vi "AnalysisConfig.vi"(8 "error in (no error)":errorcluster, 11 "AnalysisConfig":T6={"PortName"="WLAN_DUT0_ANT0", "PhyPort"=enum."Port5", "ExternalAtt"=0, "TriggerLevel"=-40, "NumberofChain"=1, "AcqLength"=0.0001, "MCSIndex"=7.0, "PhyType"=enum."OFDM", "Standard"=enum."802.11 n", "BW"=enum."20M", "TriggerSource"=enum."RIO0", "Freq"=5180000000.0, "LegacyDataRate"=enum."R1M"}) -> (0 "error out":errorcluster, 3 "AnalysisConfigCMD":string[](array[string])=["MEMory:TABLe:DELete:ALL", "ROUTe:RFSG:PORT:DELete:ALL", "TRIG:RFSA:WLAN:EDGE RISING", "TRIG:RFSA:WLAN:MQTime  5e-6", "ROUTe:RFSA:PORT:DEFine 'wlan_DUT0_ant0','Port0'", "CONF:RFSA:WLAN:CSEG:EATT:ALL 0", "TRIG:RFSA:WLAN:SOUR 'RF0'", "TRIG:RFSA:WLAN:THR 0", "CONF:RFSA:WLAN:NCH 0", "CONF:RFSA:WLAN:CSEG:PORT \"wlan_DUT0_ant0\"", "CONF:RFSA:WLAN:CSEG:FREQ:CENT 5", "CONF:RFSA:WLAN:BWID 0", "CONF:RFSA:WLAN:STAN A", "CONF:RFSA:WLAN:ALENgth 0", "CONF:RFSA:WLAN:PACK:MCS 0", "CONF:RFSA:WLAN:PHY DSSS", "CONF:RFSA:WLAN:ACT:ALL 1", "CONF:RFSA:WLAN:CSEG:POW:AUTO ON", "CONF:RFSA:WLAN:PACK:NSTS 1 ", "CONF:RFSA:WLAN:PACK:GINT LONG", "CONF:RFSA:WLAN:PACK:DMOD ALL", "CONF:RFSA:WLAN:PACK:PAYL:LENGth 1500", "CONF:RFSA:WLAN:MEAS:MOD:ENAB ON", "CONF:RFSA:WLAN:MEAS:MOD:OFDM:EST:COFF ON", "CONF:RFSA:WLAN:MEAS:MOD:OFDM:EST:IMP ON", "CONF:RFSA:WLAN:MEAS:MOD:OFDM:TRAC:AMPL OFF", "CONF:RFSA:WLAN:MEAS:MOD:OFDM:TRAC:CHAN OFF", "CONF:RFSA:WLAN:MEAS:MOD:OFDM:TRAC:TIME ON", "CONF:RFSA:WLAN:MEAS:MOD:OFDM:TRAC:PHAS NONE", "CONF:RFSA:WLAN:MEAS:MOD:AVER:COUN 50", "CONF:RFSA:WLAN:MEAS:MOD:OFDM:MSYM 16", "CONF:RFSA:WLAN:MEAS:SEM:ENAB ON ", "CONF:RFSA:WLAN:MEAS:SEM:AVER:COUN 3", "CONF:RFSA:WLAN:MEAS:SEM:SPAN:AUTO:ENAB ON", "CONF:RFSA:WLAN:MEAS:OBW:ENAB ON", "CONF:RFSA:WLAN:MEAS:OBW:AVER:COUN 3", "CONF:RFSA:WLAN:MEAS:TXP:ENAB ON", "CONF:RFSA:WLAN:MEAS:TXP:AVER:COUN 3"])   [LabVIEW 2015]
uses:
  PhyPort.ctl
  PhyType.ctl
  standard.ctl
  BW.ctl
  LegacyDataRate.ctl
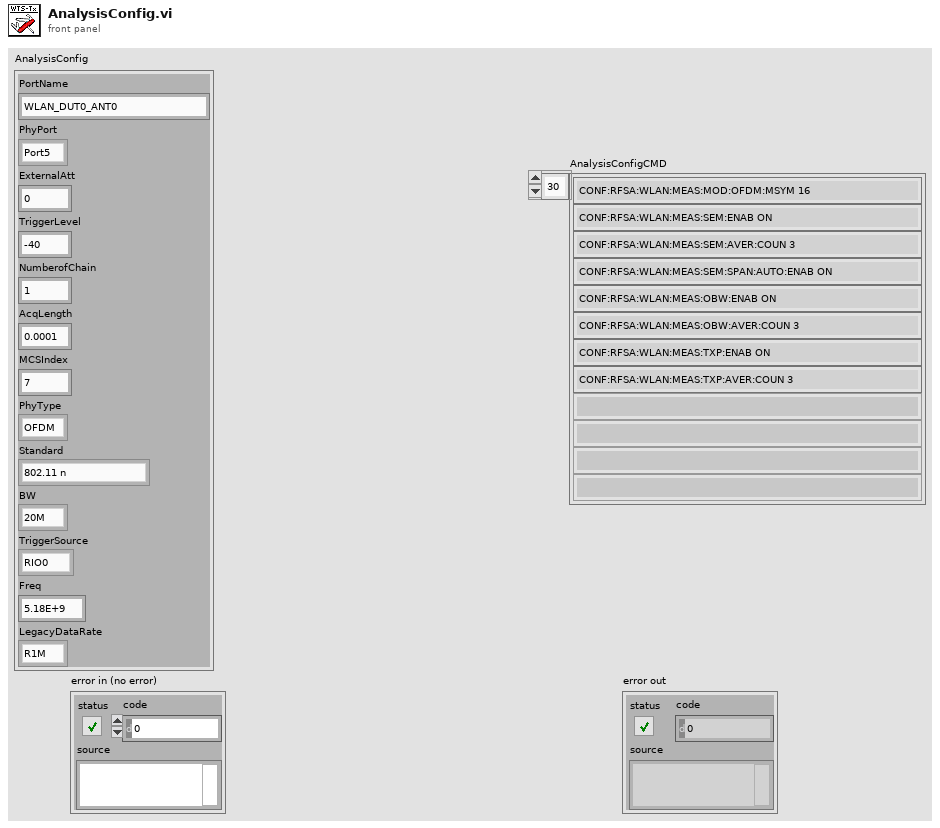
[diagram p1: front panel]
types:
  T1 = typedef "PhyPort.ctl" = enum16{"Port0", "Port1", "Port2", "Port3", "Port4", "Port5", "Port6", "Port7"}
  T2 = typedef "PhyType.ctl" = enum16{"DSSS", "OFDM", "HT", "VHT"}
  T3 = typedef "standard.ctl" = enum16{"802.11 a/g", "802.11 b/g", "802.11 g", "802.11 n", "802.11 ac"}
  T4 = typedef "BW.ctl" = enum16{"5M", "10M", "20M", "40M", "80M", "160M"}
  T5 = typedef "LegacyDataRate.ctl" = enum16{"R1M", "R2M", "R5M5", "R6M", "R9M", "R11M", "R12M", "R18M", "R24M", "R36M", "R48M", "R54M"}
  T6 = cluster{"PortName":string, "PhyPort":T1, "ExternalAtt":i32, "TriggerLevel":i32, "NumberofChain":i32, "AcqLength":dbl, "MCSIndex":dbl, "PhyType":T2, "Standard":T3, "BW":T4, "TriggerSource":enum16{"RIO0", "RIO1"}, "Freq":dbl, "LegacyDataRate":T5}
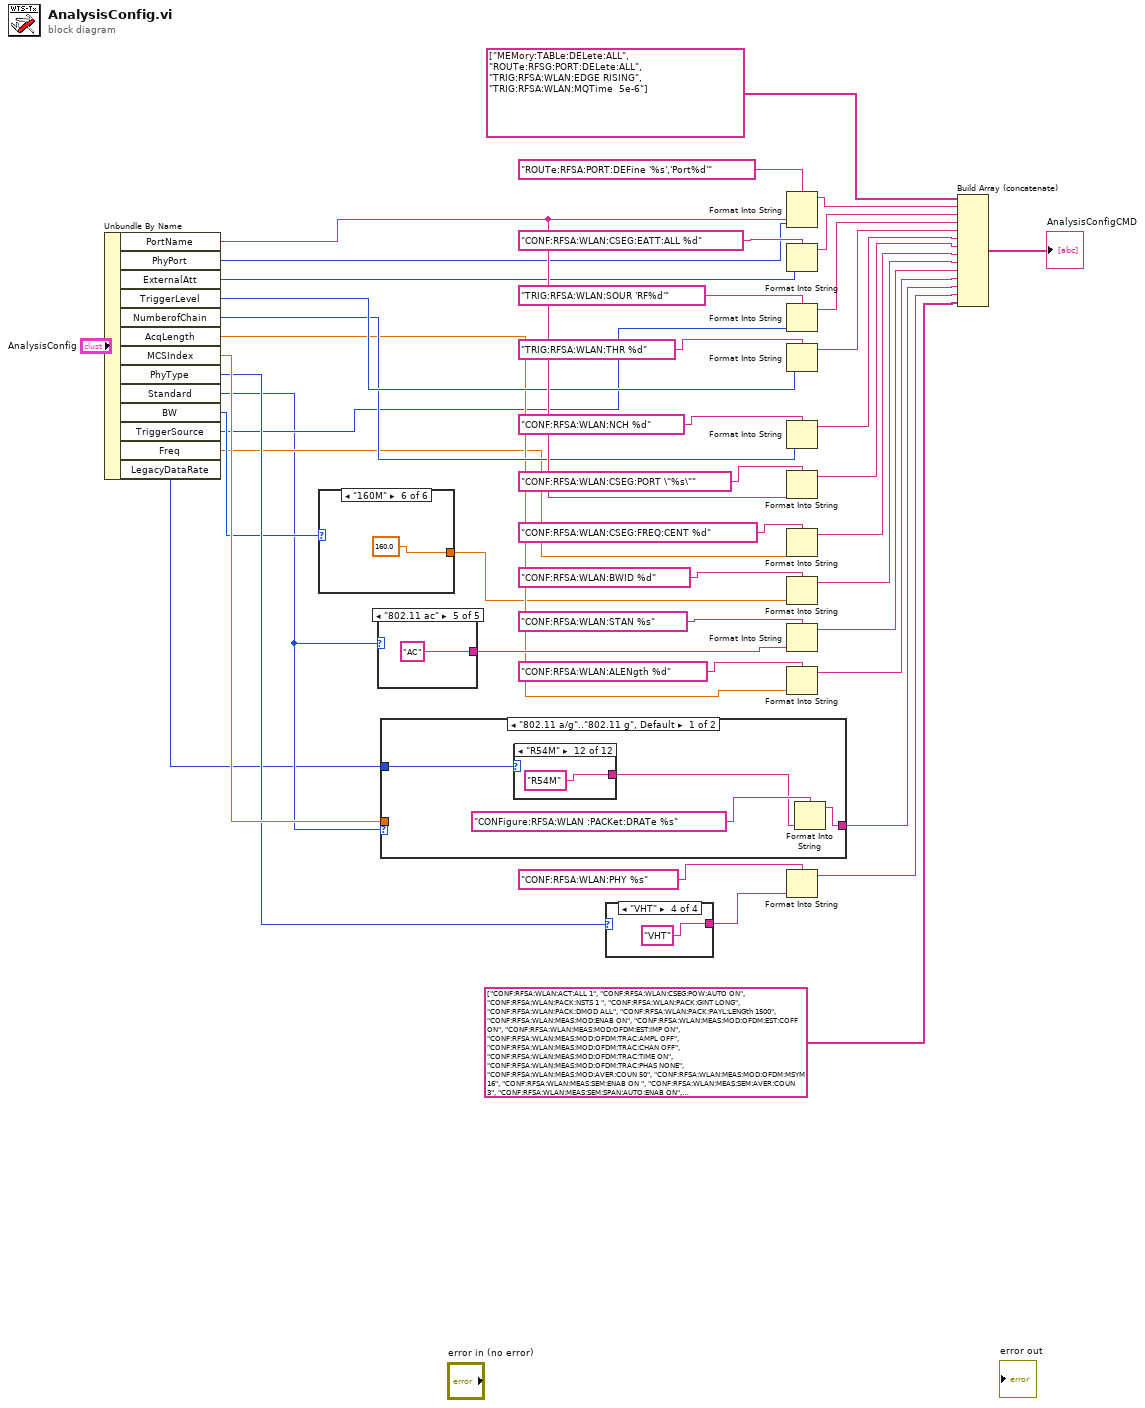
[diagram p0: block diagram]
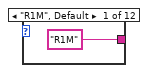
[diagram p2: hidden frame]
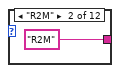
[diagram p3: hidden frame]
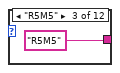
[diagram p4: hidden frame]
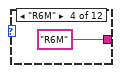
[diagram p5: hidden frame]
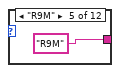
[diagram p6: hidden frame]
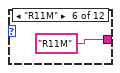
[diagram p7: hidden frame]
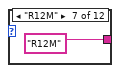
[diagram p8: hidden frame]
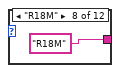
[diagram p9: hidden frame]
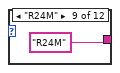
[diagram p10: hidden frame]
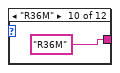
[diagram p11: hidden frame]
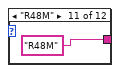
[diagram p12: hidden frame]
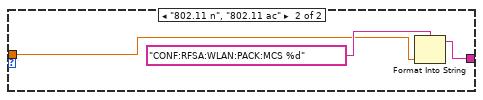
[diagram p13: hidden frame]
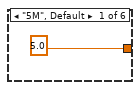
[diagram p14: hidden frame]
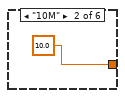
[diagram p15: hidden frame]
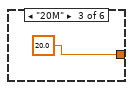
[diagram p16: hidden frame]
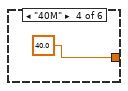
[diagram p17: hidden frame]
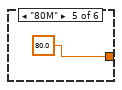
[diagram p18: hidden frame]
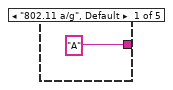
[diagram p19: hidden frame]
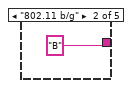
[diagram p20: hidden frame]
diagram:
  n1 = Unbundle By Name("AnalysisConfig") -> ("PortName"=w14:string, "PhyPort"=w13:T1, "ExternalAtt"=w12:i32, "TriggerLevel"=w11:i32, "NumberofChain"=w10:i32, "AcqLength"=w8:dbl, "MCSIndex"=w9:dbl, "PhyType"=w7:T2, "Standard"=w2:T3, "BW"=w6:T4, "TriggerSource"=w5:enum16{"RIO0", "RIO1"}, "Freq"=w3:dbl, "LegacyDataRate"=w1:T5)
  n2 = case shown="\"160M\"" w6 {
    tunnel: [5.0 ("Freq") 10.0 ("Freq") 20.0 ("Freq") 40.0 ("Freq") 80.0 ("Freq") 160.0 ("Freq")] -> w4
    frame "5M", Default {
    }
    frame "10M" {
    }
    frame "20M" {
    }
    frame "40M" {
    }
    frame "80M" {
    }
    frame "160M" {
    }
  }
  n3 = case shown="\"802.11 ac\"" w2 {
    tunnel: ["A" ("Standard") "B" ("Standard") "G" ("Standard") "N" ("Standard") "AC" ("Standard")] -> w16
    frame "802.11 a/g", Default {
    }
    frame "802.11 b/g" {
    }
    frame "802.11 g" {
    }
    frame "802.11 n" {
    }
    frame "802.11 ac" {
    }
  }
  n4 = case shown="\"802.11 a/g\"..\"802.11 g\", Default" w2 {
    tunnel: [w55 w72] -> w19
    tunnel: w9 -> [_ w71]
    tunnel: w1 -> [w57 _]
    frame "802.11 a/g".."802.11 g", Default {
      n5 = case shown="\"R54M\"" w57 {
        tunnel: ["R1M" "R2M" "R5M5" "R6M" "R9M" "R11M" "R12M" "R18M" "R24M" "R36M" "R48M" "R54M"] -> w56
        frame "R1M", Default {
        }
        frame "R2M" {
        }
        frame "R5M5" {
        }
        frame "R6M" {
        }
        frame "R9M" {
        }
        frame "R11M" {
        }
        frame "R12M" {
        }
        frame "R18M" {
        }
        frame "R24M" {
        }
        frame "R36M" {
        }
        frame "R48M" {
        }
        frame "R54M" {
        }
      }
      n6 = Format Into String(format string="CONFigure:RFSA:WLAN :PACKet:DRATe %s", w56) -> (resulting string=w55:string)  [unwired: 2 in, 1 out]
    }
    frame "802.11 n", "802.11 ac" {
      n7 = Format Into String(format string="CONF:RFSA:WLAN:PACK:MCS %d", w71) -> (resulting string=w72:string)  [unwired: 2 in, 1 out]
    }
  }
  n8 = case shown="\"VHT\"" w7 {
    tunnel: ["DSSS" ("PhyType") "OFDM" ("PhyType") "HT" ("PhyType") "VHT" ("PhyType")] -> w26
    frame "DSSS", Default {
    }
    frame "OFDM" {
    }
    frame "HT" {
    }
    frame "VHT" {
    }
  }
  n9 = Format Into String(format string="ROUTe:RFSA:PORT:DEFine '%s','Port%d'", w14, w13) -> (resulting string=w38:string)  [unwired: 2 in, 1 out]
  n10 = Format Into String(format string="CONF:RFSA:WLAN:CSEG:EATT:ALL %d", w12) -> (resulting string=w37:string)  [unwired: 2 in, 1 out]
  n11 = Format Into String(format string="TRIG:RFSA:WLAN:SOUR 'RF%d'", w5) -> (resulting string=w36:string)  [unwired: 2 in, 1 out]
  n12 = Format Into String(format string="TRIG:RFSA:WLAN:THR %d", w11) -> (resulting string=w35:string)  [unwired: 2 in, 1 out]
  n13 = Format Into String(format string="CONF:RFSA:WLAN:NCH %d", w10) -> (resulting string=w25:string)  [unwired: 2 in, 1 out]
  n14 = Format Into String(format string="CONF:RFSA:WLAN:CSEG:PORT \"%s\"", w14) -> (resulting string=w24:string)  [unwired: 2 in, 1 out]
  n15 = Format Into String(format string="CONF:RFSA:WLAN:CSEG:FREQ:CENT %d", w3) -> (resulting string=w23:string)  [unwired: 2 in, 1 out]
  n16 = Format Into String(format string="CONF:RFSA:WLAN:BWID %d", w4) -> (resulting string=w22:string)  [unwired: 2 in, 1 out]
  n17 = Format Into String(format string="CONF:RFSA:WLAN:STAN %s", w16) -> (resulting string=w21:string)  [unwired: 2 in, 1 out]
  n18 = Format Into String(format string="CONF:RFSA:WLAN:ALENgth %d", w8) -> (resulting string=w20:string)  [unwired: 2 in, 1 out]
  n19 = Format Into String(format string="CONF:RFSA:WLAN:PHY %s", w26) -> (resulting string=w18:string)  [unwired: 2 in, 1 out]
  n20 = Build Array (concatenate)(string[] ["MEMory:TABLe:DELete:ALL", "ROUTe:RFSG:PORT:DELete:ALL", "TRIG:RFSA:WLAN:EDGE RISING", "TRIG:RFSA:WLAN:MQTime  5e-6"], w38, w37, w36, w35, w25, w24, w23, w22, w21, w20, w19, w18, string[] ["CONF:RFSA:WLAN:ACT:ALL 1", "CONF:RFSA:WLAN:CSEG:POW:AUTO ON", "CONF:RFSA:WLAN:PACK:NSTS 1 ", "CONF:RFSA:WLAN:PACK:GINT LONG", "CONF:RFSA:WLAN:PACK:DMOD ALL", "CONF:RFSA:WLAN:PACK:PAYL:LENGth 1500", "CONF:RFSA:WLAN:MEAS:MOD:ENAB ON", "CONF:RFSA:WLAN:MEAS:MOD:OFDM:EST:COFF ON", "CONF:RFSA:WLAN:MEAS:MOD:OFDM:EST:IMP ON", "CONF:RFSA:WLAN:MEAS:MOD:OFDM:TRAC:AMPL OFF", "CONF:RFSA:WLAN:MEAS:MOD:OFDM:TRAC:CHAN OFF", "CONF:RFSA:WLAN:MEAS:MOD:OFDM:TRAC:TIME ON", "CONF:RFSA:WLAN:MEAS:MOD:OFDM:TRAC:PHAS NONE", "CONF:RFSA:WLAN:MEAS:MOD:AVER:COUN 50", "CONF:RFSA:WLAN:MEAS:MOD:OFDM:MSYM 16", "CONF:RFSA:WLAN:MEAS:SEM:ENAB ON ", "CONF:RFSA:WLAN:MEAS:SEM:AVER:COUN 3", "CONF:RFSA:WLAN:MEAS:SEM:SPAN:AUTO:ENAB ON", "CONF:RFSA:WLAN:MEAS:OBW:ENAB ON", "CONF:RFSA:WLAN:MEAS:OBW:AVER:COUN 3", "CONF:RFSA:WLAN:MEAS:TXP:ENAB ON", "CONF:RFSA:WLAN:MEAS:TXP:AVER:COUN 3", "*OPC?", "INIT:RFSA:WLAN:RES1"]) -> (→"AnalysisConfigCMD":string[])
